vi "VI_principal.vi"() -> ()   [LabVIEW 2024]
uses:
  <vilib>/LabVIEW Open Source Project/Epoch Date & Time/epoch.UNIX/Epoch.UNIX.lvclass
panel:
  in  "Tab Control":enum32{"Fase A", "Fase B", "Fase C"}(tab)
  out "Fase A":waveform(dbl)
  out "Potência A":waveform(dbl)(graph)
  out "Fase B":waveform(dbl)
  out "Potência B":waveform(dbl)(graph)
  out "Fase C":waveform(dbl)
  out "Potência C":waveform(dbl)(graph)
  in  "stop":bool
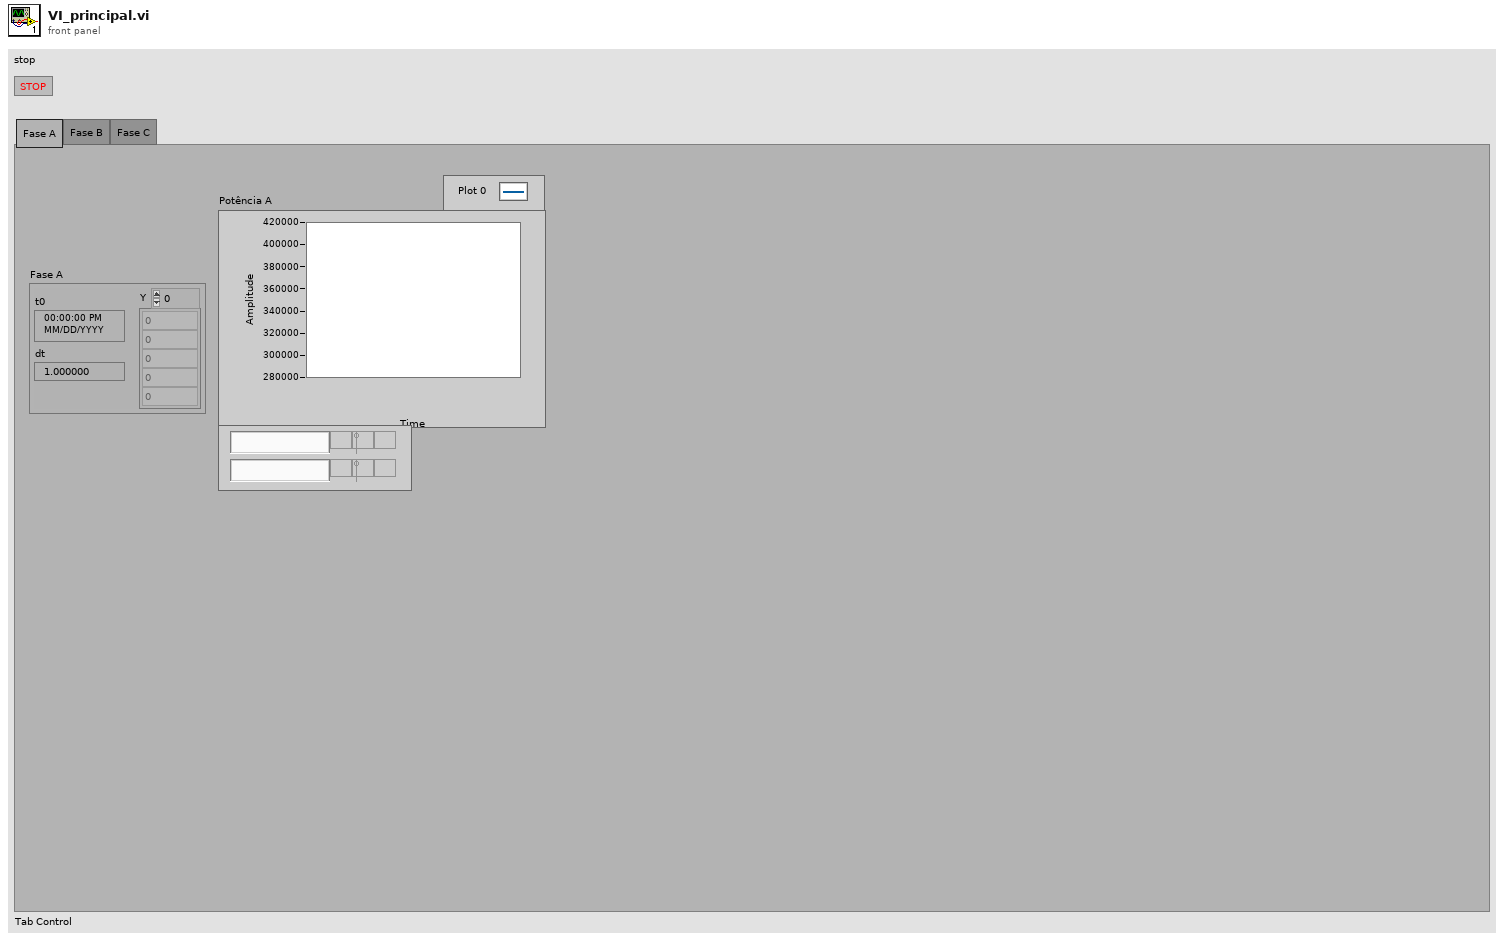
[diagram p1: front panel]
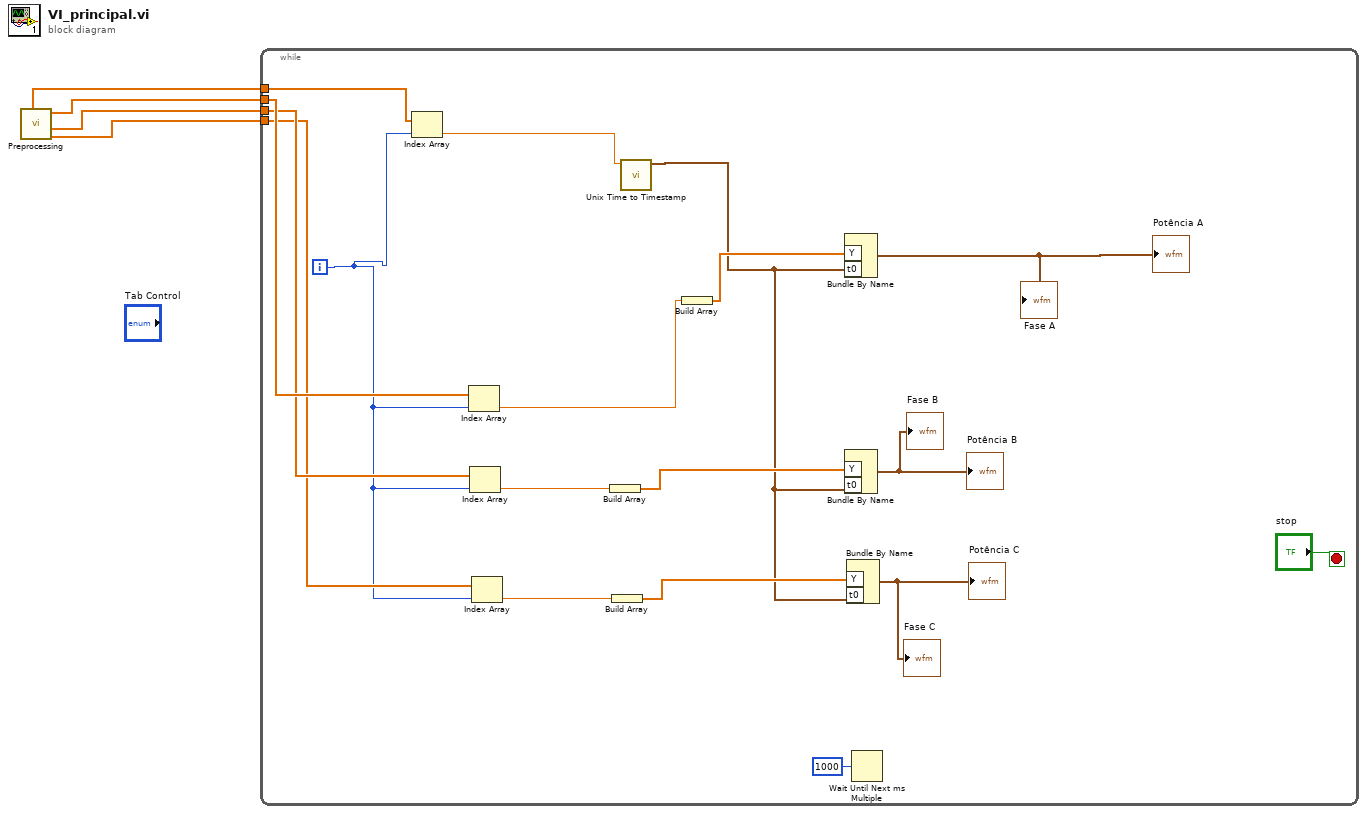
[diagram p0: block diagram]
diagram:
  n1 = call "Preprocessing.vi"() -> ("Potência Ativa C"=w1:dbl[], "Potência Ativa B"=w2:dbl[], "Potência instantänea A"=w3:dbl[], "Timestamp"=w4:dbl[])  [unwired: 6 out]
  n2 = while {
    tunnel: w3 -> [w22]
    tunnel: w4 -> [w21]
    tunnel: w2 -> [w14]
    tunnel: w1 -> [w9]
    i -> [w8]
    stop <- "stop" stop-if-true
    n3 = Index Array(array=w21, index=w8) -> (element=w20:dbl)
    n4 = Index Array(array=w22, index=w8) -> (element=w19:dbl)
    n5 = Index Array(array=w14, index=w8) -> (element=w13:dbl)
    n6 = Index Array(array=w9, index=w8) -> (element=w11:dbl)
    n7 = Build Array(w13) -> (w12:dbl[])
    n8 = Build Array(w11) -> (w10:dbl[])
    n9 = call <vilib>:"Unix Time to Timestamp.vi"("Unix Time (s)"=w20) -> ("Timestamp"=w7:timestamp)  [unwired: 9 in, 1 out]
    n10 = Build Array(w19) -> (w18:dbl[])
    n11 = Bundle By Name("Y"=w18, "t0"=w7) -> (→"Fase A" →"Potência A":waveform(dbl))  [unwired: 1 in]
    n12 = Bundle By Name("Y"=w12, "t0"=w7) -> (→"Potência B" →"Fase B":waveform(dbl))  [unwired: 1 in]
    n13 = Bundle By Name("Y"=w10, "t0"=w7) -> (→"Potência C" →"Fase C":waveform(dbl))  [unwired: 1 in]
    n14 = Wait Until Next ms Multiple(millisecond multiple=u32 1000) -> ()  [unwired: 1 out]
  }
